vi "test string esc unesc.vi"() -> ()   [LabVIEW 2017]
uses:
  JSONtext.lvlib
panel:
  out "jsontext escape matches lvjson":bool
  out "JSON string":string
  out "<JSON>":string caption="jsonstring escape"
  out "junk string err":errorcluster
  out "junk array ok self>self":bool
  out "gross string ok self>self":bool
  out "char by char failed":cluster{"in":string, "out":string}[](array[cluster])
  out "char by char check":bool
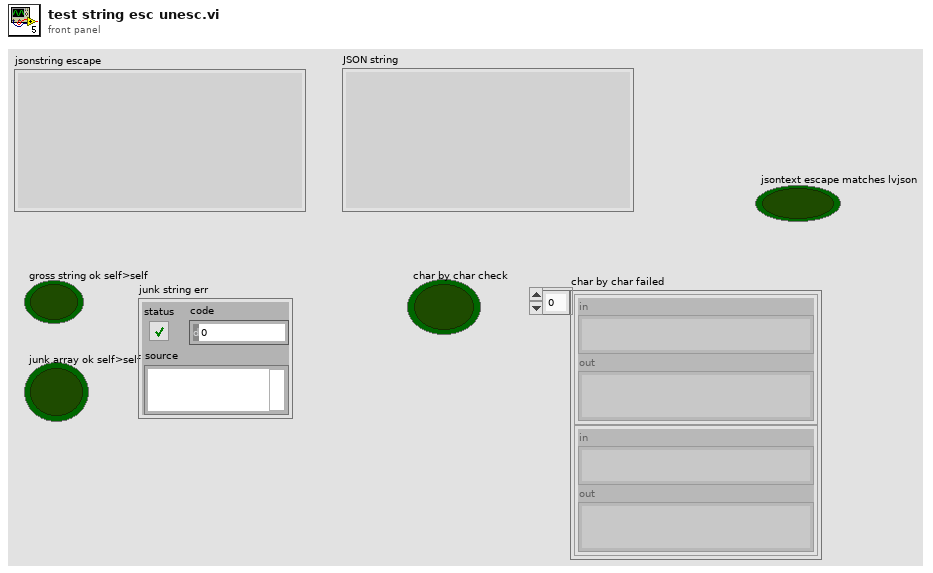
[diagram p1: front panel]
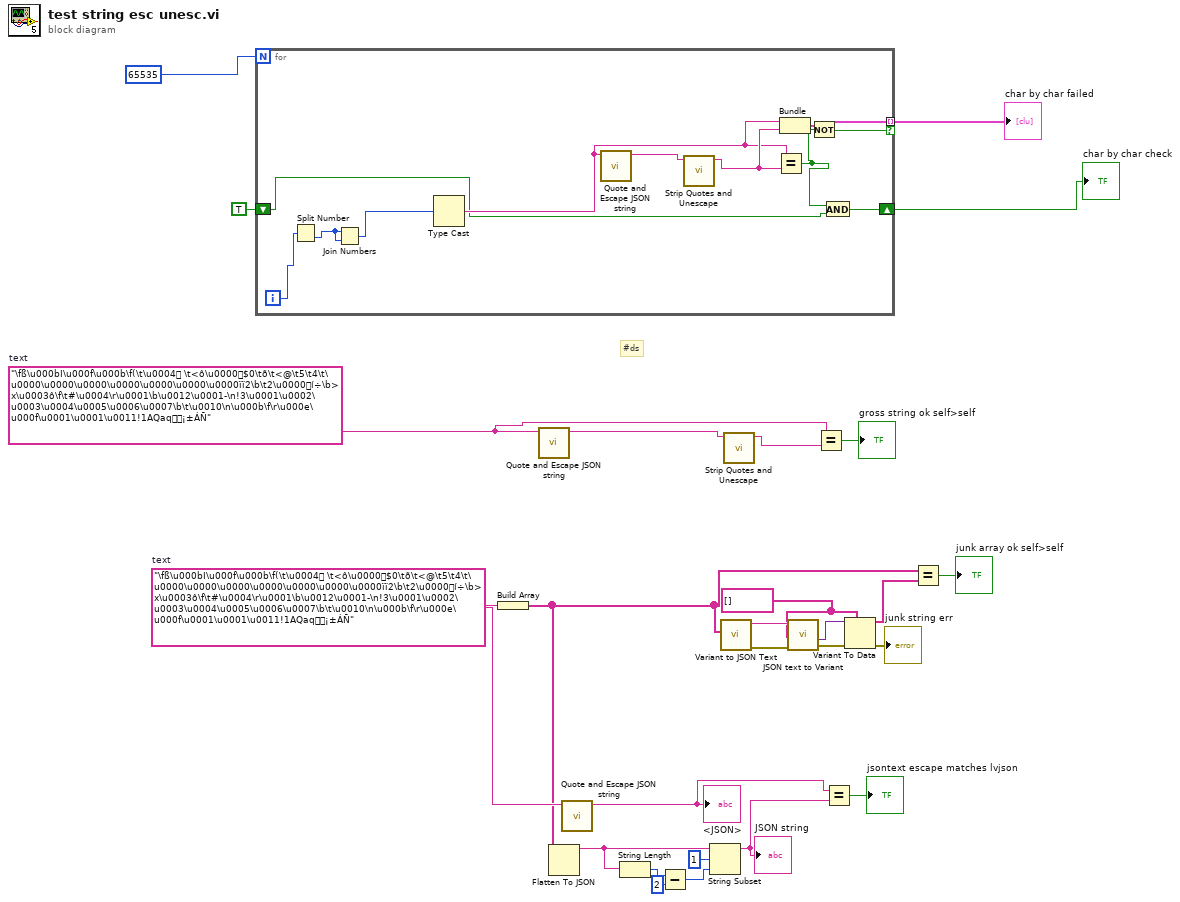
[diagram p0: block diagram]
diagram:
  w13 = string[] []
  w10 = "\fß\u000bI\u000f\u000b\f(\t\u0004 \t<ô\u0000$0\tð\t<@\t5\t4\t\u0000\u0000\u0000\u0000\u0000\u0000\u0000ïï2\b\t2\u0000í÷\b> x\u0003ô\f\t#\u0004\r\u0001\b\u0012\u0001-\n!3\u0001\u0002\u0003\u0004\u0005\u0006\u0007\b\t\u0010\n\u000b\f\r\u000e\u000f\u0001\u0001\u0011!1AQaq¡±ÁÑ"  # text
  w20 = "\fß\u000bI\u000f\u000b\f(\t\u0004 \t<ô\u0000$0\tð\t<@\t5\t4\t\u0000\u0000\u0000\u0000\u0000\u0000\u0000ïï2\b\t2\u0000í÷\b> x\u0003ô\f\t#\u0004\r\u0001\b\u0012\u0001-\n!3\u0001\u0002\u0003\u0004\u0005\u0006\u0007\b\t\u0010\n\u000b\f\r\u000e\u000f\u0001\u0001\u0011!1AQaq¡±ÁÑ"  # text
  # "#ds"
  n1 = for {
    N: 65535 -> [_]
    tunnel: [w35] -> w26 mode=indexing if=w36
    shift-right: [w31] -> w23
    shift-left: TRUE -> [w30]
    i -> [w29]
    n2 = Split Number(x=w29) -> (lo(x)=w28:u16)  [unwired: 1 out]
    n3 = Join Numbers(hi=w28, lo=w28) -> ((hi.lo)=w27:u32)
    n4 = Type Cast(x=w27) -> (*(type *) &x=w33:string)  [unwired: 1 in]
    n5 = call "Quote and Escape JSON string.vi"("Plain Text"=w33) -> ("<JSON>"=w37:string)  [unwired: 10 in]
    n6 = call "Strip Quotes and Unescape.vi"("String"=w37) -> ("result string"=w34:string)  [unwired: 9 in, 1 out]
    n7 = Equal?(x=w33, y=w34) -> (x = y?=w32:bool)
    n8 = Bundle(w33, "result string"=w34) -> (w35:cluster{string, "result string":string})  [unwired: 1 in]
    n9 = Not(x=w32) -> (.not. x?=w36:bool)
    n10 = And(x=w32, y=w30) -> (x .and. y?=w31:bool)
  }
  "char by char check" <- w23
  "char by char failed" <- w26
  n11 = Build Array(w10) -> (w9:string[])
  n12 = call "Quote and Escape JSON string.vi"("Plain Text"=w20) -> ("<JSON>"=w21:string)  [unwired: 10 in]
  n13 = Flatten To JSON(anything=w9) -> (JSON string=w8:string)  [unwired: 2 in, 1 out]
  n14 = call "Quote and Escape JSON string.vi"("Plain Text"=w10) -> ("<JSON>"=w2:string)  [unwired: 10 in]
  "<JSON>" <- w2
  n15 = String Length(string=w8) -> (length=w7:i32)
  n16 = Subtract(x=w7, y=2) -> (x-y=w5:i32)
  n17 = String Subset(string=w8, offset (0)=1, length (rest)=w5) -> (substring=w3:string)
  "JSON string" <- w3
  n18 = call "Variant to JSON Text.vi"("Variant"=w9) -> ("error out"=w17:errorcluster, "<JSON>"=w18:string)  [unwired: 8 in, 1 out]
  n19 = call "Strip Quotes and Unescape.vi"("String"=w21) -> ("result string"=w22:string)  [unwired: 9 in, 1 out]
  n20 = call "JSON text to Variant.vi"("error in (no error)"=w17, "Data Type"=w13, "JSON"=w18) -> ("error out"=w15:errorcluster, "Variant out"=w16:variant)  [unwired: 7 in]
  n21 = Equal?(x=w20, y=w22) -> (x = y?=→"gross string ok self>self":bool)
  n22 = Equal?(x=w2, y=w3) -> (x = y?=→"jsontext escape matches lvjson":bool)
  n23 = Variant To Data(error in=w15, type=w13, Variant=w16) -> (data=w12:string[], error out=→"junk string err":errorcluster)
  n24 = Equal?(x=w9, y=w12) -> (x = y?=→"junk array ok self>self":bool)
